vi "培训1#.vi"() -> ()   [LabVIEW 2019]
panel:
  out "数组 4":i32[](array[numeric])
  out "数组 2":dbl[](array[numeric])=[1.0, 2.0, 3.0]
  out "数值 7":dbl
  in  "y":dbl
  in  "x":dbl
  out "数组3 2":dbl[][](array[numeric])
  out "数组":dbl[](array[numeric])
  in  "数值 6":dbl
  out "数值 5":dbl=30300.0
  out "数值 4":dbl
  in  "数值 3":dbl
  out "数值 2":dbl
  in  "数值":dbl
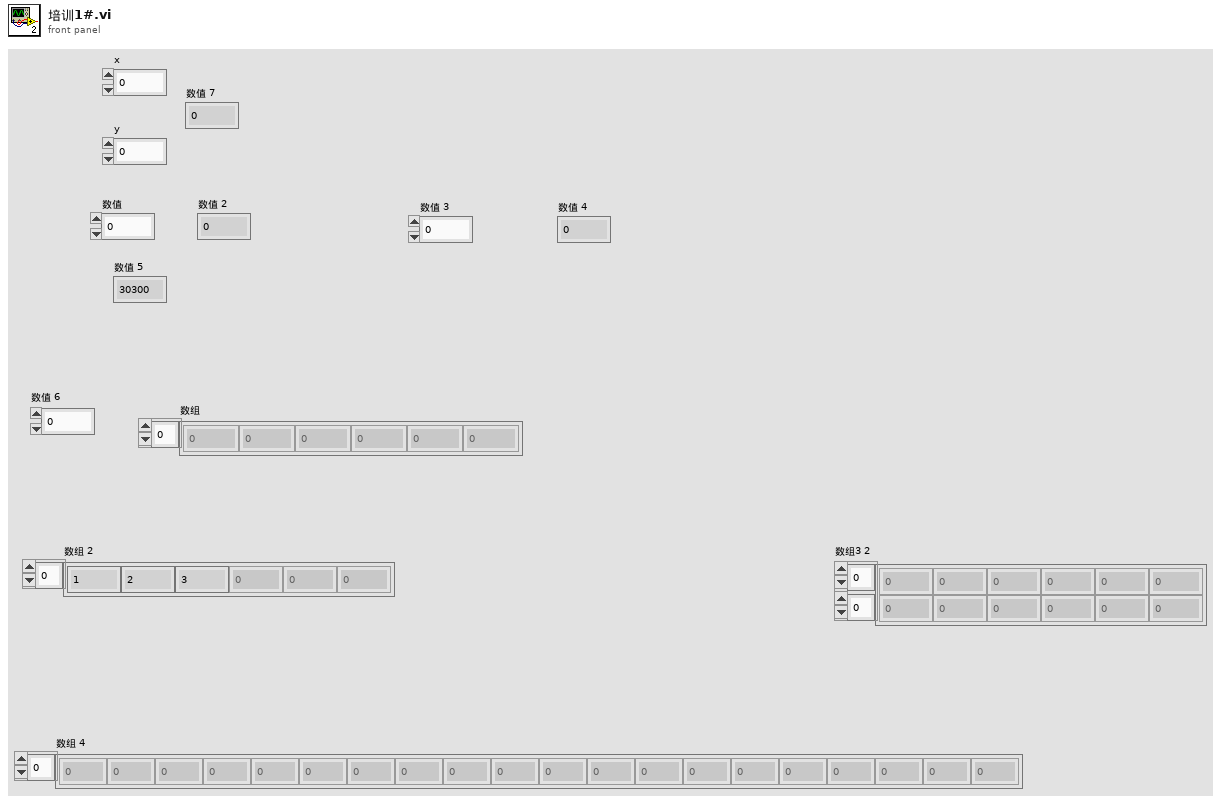
[diagram p1: front panel]
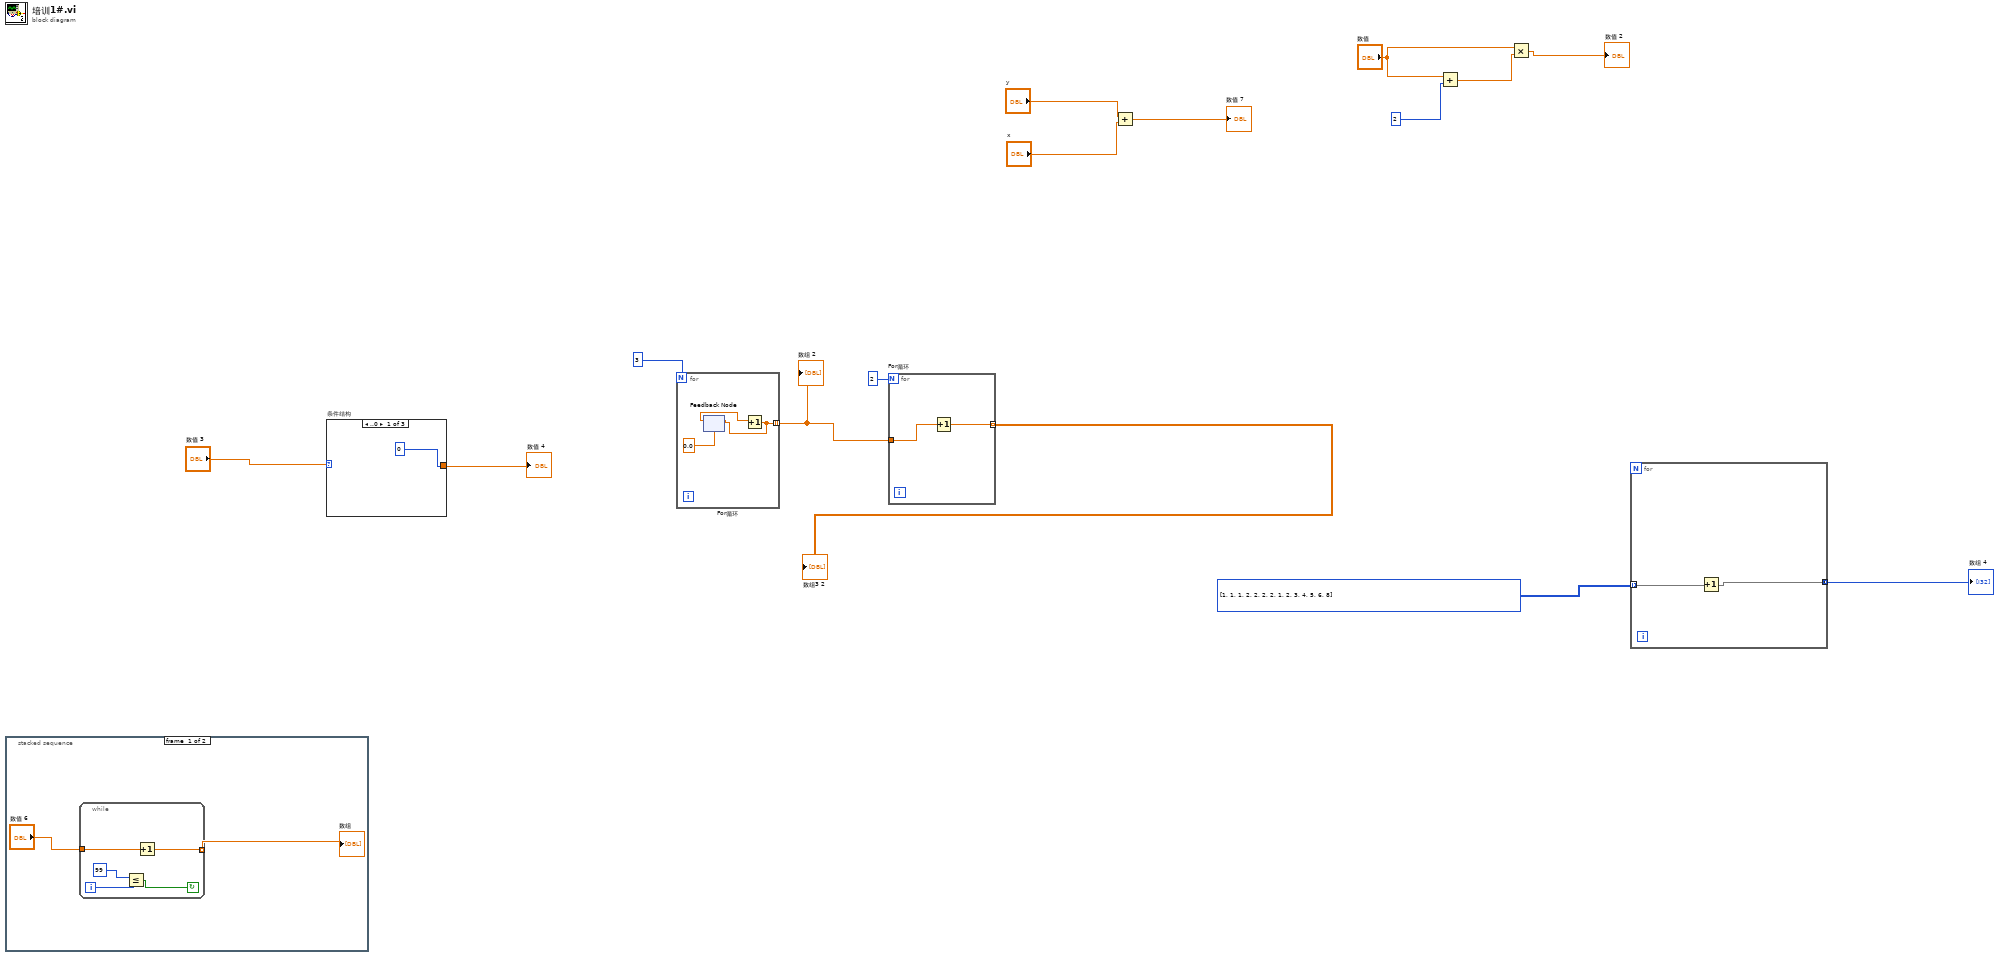
[diagram p0: block diagram]
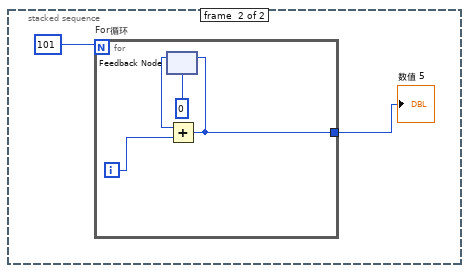
[diagram p2: hidden frame]
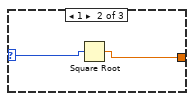
[diagram p3: hidden frame]
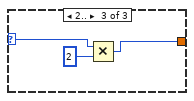
[diagram p4: hidden frame]
diagram:
  n1 = stacked-sequence {
    frame #0 {
      n2 = while {
        tunnel: "数值 6" -> [w19]
        tunnel: [w18] -> w16 mode=indexing
        i -> [w22]
        stop <- w20 continue-if-true
        n3 = Less Or Equal?(x=99, y=w22) -> (x <= y?=w20:bool)
        n4 = Increment(x=w19) -> (x+1=w18:dbl)
      }
      "数组" <- w16
    }
    frame #1 {
      n5 = for "For循环" {
        N: 101 -> [_]
        tunnel: [w27] -> w24
        i -> [w26]
        n6 = feedback #1(0) -> (w28:i32)
        n7 = Add(x=w28, y=w26) -> (x+y=w27:i32)
        n8 = feedback-in #1(w27) -> ()
      }
      "数值 5" <- w24
    }
  }
  n9 = case "条件结构" shown="..0" "数值 3" {
    selector: "数值 3" -> [_ w31 w34]
    tunnel: [0 w30 w32] -> w15
    frame ..0 {
    }
    frame 1 {
      n10 = Square Root(x=w31) -> (sqrt(x)=w30:dbl)
    }
    frame 2.. {
      n11 = Multiply(x=w34, y=2) -> (x*y=w32:i32)
    }
  }
  "数值 4" <- w15
  n12 = for "For循环" {
    N: 3 -> [_]
    tunnel: [w35] -> w12 mode=indexing
    n13 = feedback #2(0.0) -> (w36:dbl)
    n14 = Increment(x=w36) -> (x+1=w35:dbl)
    n15 = feedback-in #2(w35) -> ()
  }
  "数组 2" <- w12
  n16 = for "For循环" {
    N: 2 -> [_]
    tunnel: w12 -> [w39]
    tunnel: [w38] -> w11 mode=indexing
    n17 = Increment(x=w39) -> (x+1=w38:dbl[])
  }
  "数组3 2" <- w11
  n18 = Add(x="y", y="x") -> (x+y=→"数值 7":dbl)
  n19 = Add(x="数值", y=2) -> (x+y=w7:dbl)
  n20 = Multiply(x="数值", y=w7) -> (x*y=→"数值 2":dbl)
  n21 = for {
    tunnel: [w41] -> w10 mode=concatenating
    tunnel: i32[][] [[1, 1, 1, 2, 2, 2, 2], [1, 2, 3, 4, 5, 6, 8]] -> [w40] mode=indexing
    n22 = Increment(x=w40) -> (x+1=w41:i32[])
  }
  "数组 4" <- w10
